vi "Configure Analog Alarm Parameters 2.vi"(0 "VISA resource name":refnum<visa-resource-name>, 1 "Unit Address (1)":u8=1, 2 "Alarm Number (1)":u16=1 min=1 max=8, 5 "Display Delay (0)":u32 max=1800000000, 7 "Reference Value (0)":i32 min=-10000 max=10000, 9 "Alarm Inhibit  (False:Disable)":bool, 11 "error in (no error)":errorcluster, 12 "Alarm Blocking Mode (False: Disable)":bool) -> (4 "VISA resource name out":refnum<visa-resource-name>, 15 "error out":errorcluster)   [LabVIEW 2014, in "Eurotherm 35xx Series.lvlib"]
doc: "This VI Configure parameters of selected analog alarm (part 2)."
uses:
  <instrlib>/Eurotherm 35xx Series/Eurotherm 35xx Series.lvlib
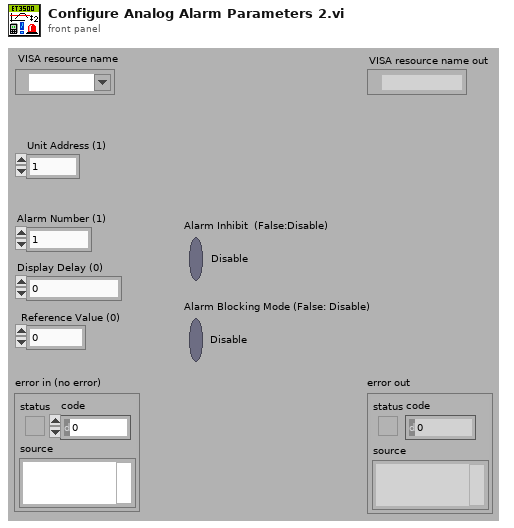
[diagram p1: front panel]
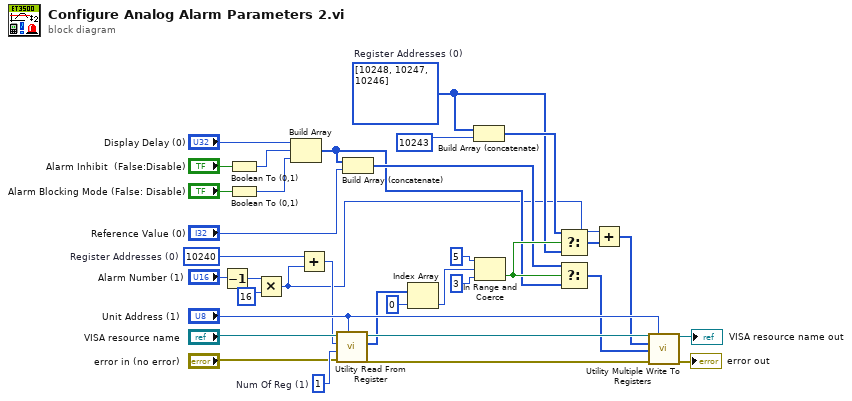
[diagram p0: block diagram]
diagram:
  w6 = u16[] [10248, 10247, 10246]  # Register Addresses (0)
  w25 = u16 1  # Num Of Reg (1)
  w31 = u16 10240  # Register Addresses (0)
  n1 = Decrement(x="Alarm Number (1)") -> (x-1=w33:u16)
  n2 = Boolean To (0,1)(Boolean="Alarm Inhibit  (False:Disable)") -> (0, 1=w11:i16)
  n3 = Boolean To (0,1)(Boolean="Alarm Blocking Mode (False: Disable)") -> (0, 1=w10:i16)
  n4 = Multiply(x=w33, y=u16 16) -> (x*y=w1:u16)
  n5 = Build Array("Display Delay (0)", w11, w10) -> (w5:u32[])
  n6 = Add(x=w31, y=w1) -> (x+y=w26:u16)
  n7 = call <instrlib>:"Utility Read From Register.vi"("Unit Address (1)"="Unit Address (1)", "error in (no error)"="error in (no error)", "Num Of Reg (1)"=w25, "Register Address (0)"=w26, "VISA resource name"="VISA resource name") -> ("error out"=w22:errorcluster, "Data"=w21:i16[], "VISA resource name out"=w23:refnum<visa-resource-name>)  [unwired: 4 in]
  n8 = Build Array (concatenate)(w5, "Reference Value (0)") -> (w7:u32[])
  n9 = Index Array(array=w21, index=0) -> (element=w16:i16)
  n10 = Build Array (concatenate)(w6, 10243 ("y")) -> (w8:i32[])
  n11 = In Range and Coerce(upper limit=i16 5, x=w16, lower limit=i16 3) -> (In Range?=w15:bool)  [unwired: 1 out]
  n12 = Select(t=w8, s=w15, f=w6) -> (s? t:f=w3:i32[])
  n13 = Select(t=w7, s=w15, f=w5) -> (s? t:f=w4:u32[])
  n14 = Add(x=w1, y=w3) -> (x+y=w2:i32[])
  n15 = call <instrlib>:"Utility Multiple Write To Registers.vi"("VISA resource name"=w23, "Unit Address (1)"="Unit Address (1)", "Registers Addresses (0)"=w2, "Data (0)"=w4, "error in (no error)"=w22) -> ("VISA resource name out"=→"VISA resource name out":refnum<visa-resource-name>, "error out"=→"error out":errorcluster)  [unwired: 9 in]
